vi "Periodic Tasks.vi"(8 "error in":errorcluster) -> ()   [LabVIEW 2018]
doc: "This VI runs in parallel to other robot code. It can contain as many user-defined periodic loops as you need. These can carry out PID or other sorts of timed response."
uses:
  <vilib>/Rock Robotics/WPI/Utilities/WPI_GetSetVariantRefNum.vi
  Robot Global Data.vi
panel:
  out "Cargo Stop Current":dbl=10.0 format="%#_13g"
  out "Stop the grabber":bool
  out "Solenoid Voltage":dbl
  out "Input Voltage":dbl
  out "Compressor current (A)":dbl
  out "all currents (A)":dbl[](array[numeric]) caption="0\n1\n2\n3\n4\n5\n6\n7\n8\n9\n10\n11\n12\n13\n14\n15"
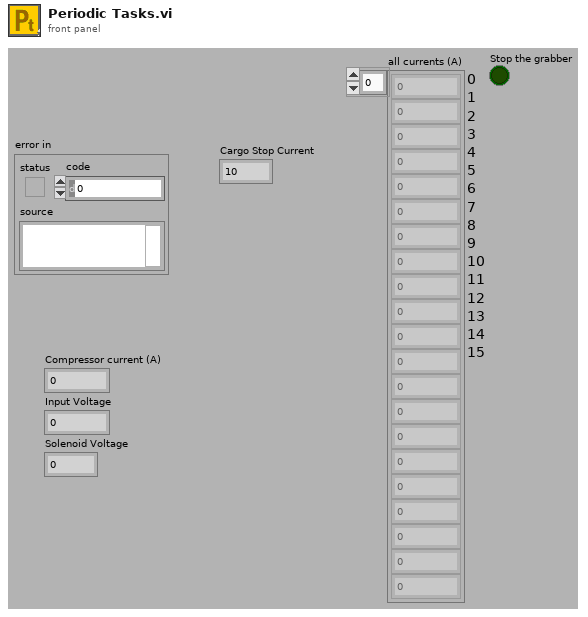
[diagram p1: front panel]
types:
  T1 = typedef "WPI_JoystickDevRef.ctl" = cluster{"Device":T2}
  T2 = typedef "WPI_JoystickDeviceEnum.ctl" = enum16{"USB 0", "USB 1", "USB 2", "USB 3", "USB 4", "USB 5"}
  T3 = cluster{"JoystickDevRef":T1, "JoystickDevRef":T1}
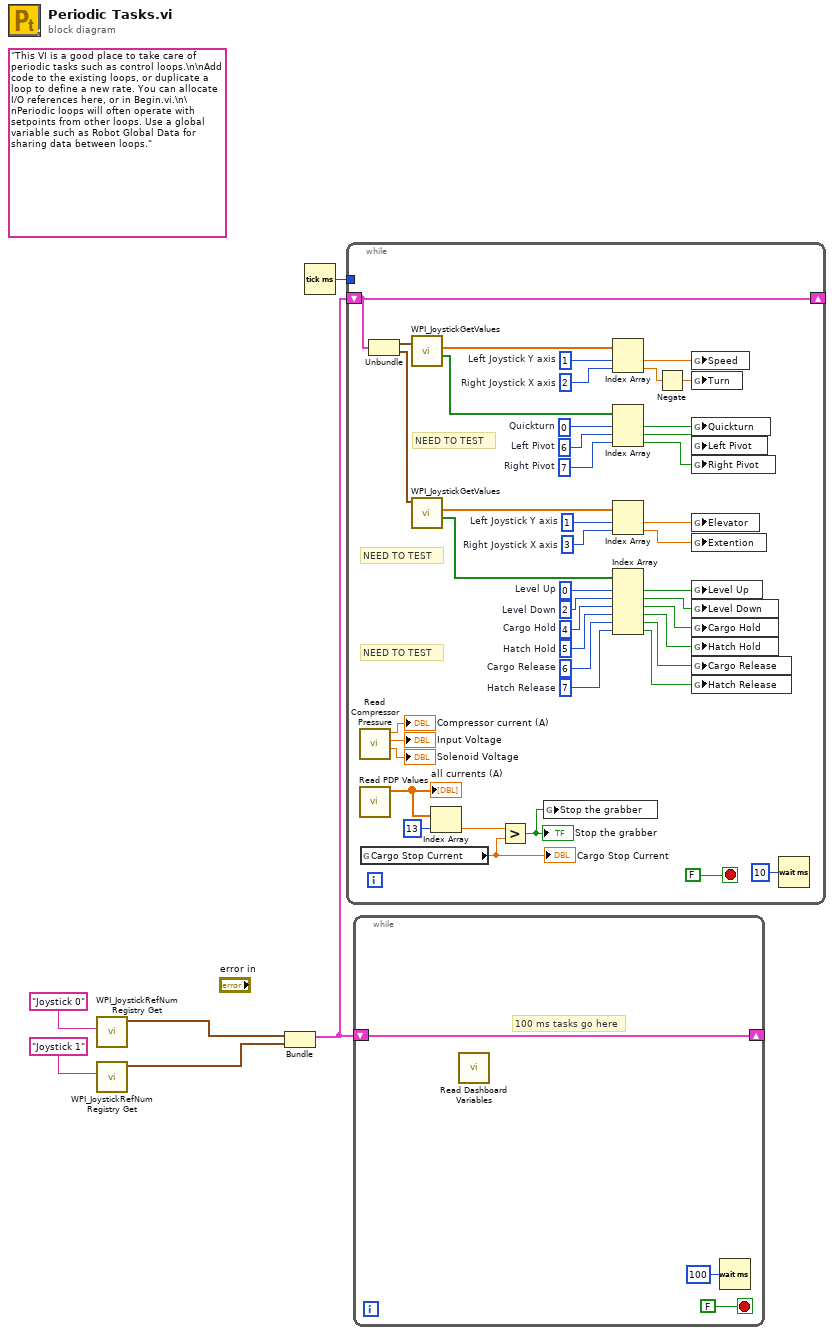
[diagram p0: block diagram]
diagram:
  (unwired) "This VI is a good place to take care of periodic tasks such as control loops.\n\nAdd code to the existing loops, or duplicate a loop to define a new rate. You can allocate I/O references here, or in Begin.vi.\n\nPeriodic loops will often operate with setpoints from other loops. Use a global variable such as Robot Global Data for sharing data between loops."
  n1 = call <vilib>:"WPI_JoystickRefNum Registry Get.vi"("refnum name"="Joystick 0") -> ("JoystickDevRef"=w3:T1)  [unwired: 1 in, 9 out]
  n2 = call <vilib>:"WPI_JoystickRefNum Registry Get.vi"("refnum name"="Joystick 1") -> ("JoystickDevRef"=w1:T1)  [unwired: 1 in, 9 out]
  n3 = Bundle("JoystickDevRef"=w3, "JoystickDevRef"=w1) -> (w2:T3)  [unwired: 1 in]
  n4 = Tick Count (ms)() -> (millisecond timer value=w5:u32)
  n5 = while {
    shift-right: [w44] -> _
    shift-left: w2 -> [w44]
    tunnel: w5 -> [_]
    stop <- FALSE stop-if-true
    w13 = 7  # Hatch Release
    w14 = 6  # Cargo Release
    w15 = 5  # Hatch Hold
    w16 = 4  # Cargo Hold
    w17 = 2  # Level Down
    w18 = 0  # Level Up
    w22 = 3  # Right Joystick X axis
    w23 = 1  # Left Joystick Y axis
    w26 = 7  # Right Pivot
    w27 = 6  # Left Pivot
    w28 = 0  # Quickturn
    w38 = 2  # Right Joystick X axis
    w39 = 1  # Left Joystick Y axis
    # "NEED TO TEST"
    # "NEED TO TEST"
    # "NEED TO TEST"
    n6 = call "Read Compressor Pressure.vi"() -> ("Solenoid Voltage"=→"Solenoid Voltage":dbl, "Input Voltage"=→"Input Voltage":dbl, "Compressor current (A)"=→"Compressor current (A)":dbl)  [unwired: 9 in]
    n7 = call "Read PDP Values.vi"() -> ("all currents (A)"=w30:dbl[])  [unwired: 11 in]
    "all currents (A)" <- w30
    n8 = global read "Robot Global Data.vi" "Cargo Stop Current"() -> (w19:dbl)
    "Cargo Stop Current" <- w19
    n9 = Unbundle(w44) -> ("JoystickDevRef"=w43:T1, "JoystickDevRef"=w40:T1)
    n10 = call <vilib>:"WPI_JoystickGetValues.vi"("JoystickDevRef"=w43) -> ("Buttons"=w46:bool[], "Axes"=w48:dbl[])  [unwired: 6 in, 3 out]
    n11 = call <vilib>:"WPI_JoystickGetValues.vi"("JoystickDevRef"=w40) -> ("Buttons"=w42:bool[], "Axes"=w41:dbl[])  [unwired: 6 in, 3 out]
    n12 = Index Array(array=w30, index=13) -> (element=w32:dbl)
    n13 = Greater?(x=w32, y=w19) -> (0:w29:bool)
    "Stop the grabber" <- w29
    n14 = global write "Robot Global Data.vi" "Stop the grabber"(w29) -> ()
    n15 = Index Array(array=w48, index #1=w39, index #2=w38) -> (element #1=w37:dbl, element #2=w36:dbl)
    n16 = Index Array(array=w46, index #1=w28, index #2=w27, index #3=w26) -> (element #1=w45:bool, element #2=w25:bool, element #3=w24:bool)
    n17 = Index Array(array=w41, index #1=w23, index #2=w22) -> (element #1=w21:dbl, element #2=w20:dbl)
    n18 = Index Array(array=w42, index #1=w18, index #2=w17, index #3=w16, index #4=w15, index #5=w14, index #6=w13) -> (element #1=w12:bool, element #2=w11:bool, element #3=w10:bool, element #4=w9:bool, element #5=w8:bool, element #6=w7:bool)
    n19 = Negate(x=w36) -> (-x=w47:dbl)
    n20 = global write "Robot Global Data.vi" "Speed"(w37) -> ()
    n21 = global write "Robot Global Data.vi" "Turn"(w47) -> ()
    n22 = global write "Robot Global Data.vi" "Quickturn"(w45) -> ()
    n23 = global write "Robot Global Data.vi" "Left Pivot"(w25) -> ()
    n24 = global write "Robot Global Data.vi" "Right Pivot"(w24) -> ()
    n25 = global write "Robot Global Data.vi" "Elevator"(w21) -> ()
    n26 = global write "Robot Global Data.vi" "Extention"(w20) -> ()
    n27 = global write "Robot Global Data.vi" "Level Up"(w12) -> ()
    n28 = global write "Robot Global Data.vi" "Level Down"(w11) -> ()
    n29 = global write "Robot Global Data.vi" "Cargo Hold"(w10) -> ()
    n30 = global write "Robot Global Data.vi" "Hatch Hold"(w9) -> ()
    n31 = global write "Robot Global Data.vi" "Cargo Release"(w8) -> ()
    n32 = global write "Robot Global Data.vi" "Hatch Release"(w7) -> ()
    n33 = Wait (ms)(milliseconds to wait=u32 10) -> ()  [unwired: 1 out]
  }
  n34 = while {
    shift-right: [w51] -> _
    shift-left: w2 -> [w51]
    stop <- FALSE stop-if-true
    # "100 ms tasks go here"
    n35 = call "Read Dashboard Variables.vi"() -> ()  [unwired: 12 in]
    n36 = Wait (ms)(milliseconds to wait=u32 100) -> ()  [unwired: 1 out]
  }
